vi "Lixiang's SRAM SEU mapping.vi"() -> ()   [LabVIEW 2015]
panel:
  out "subarray":i32[][](array[numeric])
  out "Array 2":i32[][](array[numeric])
  out "Intensity Graph 3":i32[][](graph)
  out "Intensity Graph 2":i32[][](graph)
  out "Intensity Graph":i32[][](graph)
  out "output array 3":bool[][](array[boolean])
  out "output array 2":bool[][](array[boolean])
  out "output array":bool[][](array[boolean])
  out "Array":u32[](array[numeric])
  out "number of replacements":i32
  out "SEU Information":string
  out "1->0":dbl
  out "0->1":dbl
  out "SEU":dbl
  in  "Data Pattern":i32=2
  out "result string":string
  out "text":string
  # "SRAM SEU Data Processing Program"
  # "Regular Model"
  # "0: 00  \n1: 10\n2: 11"
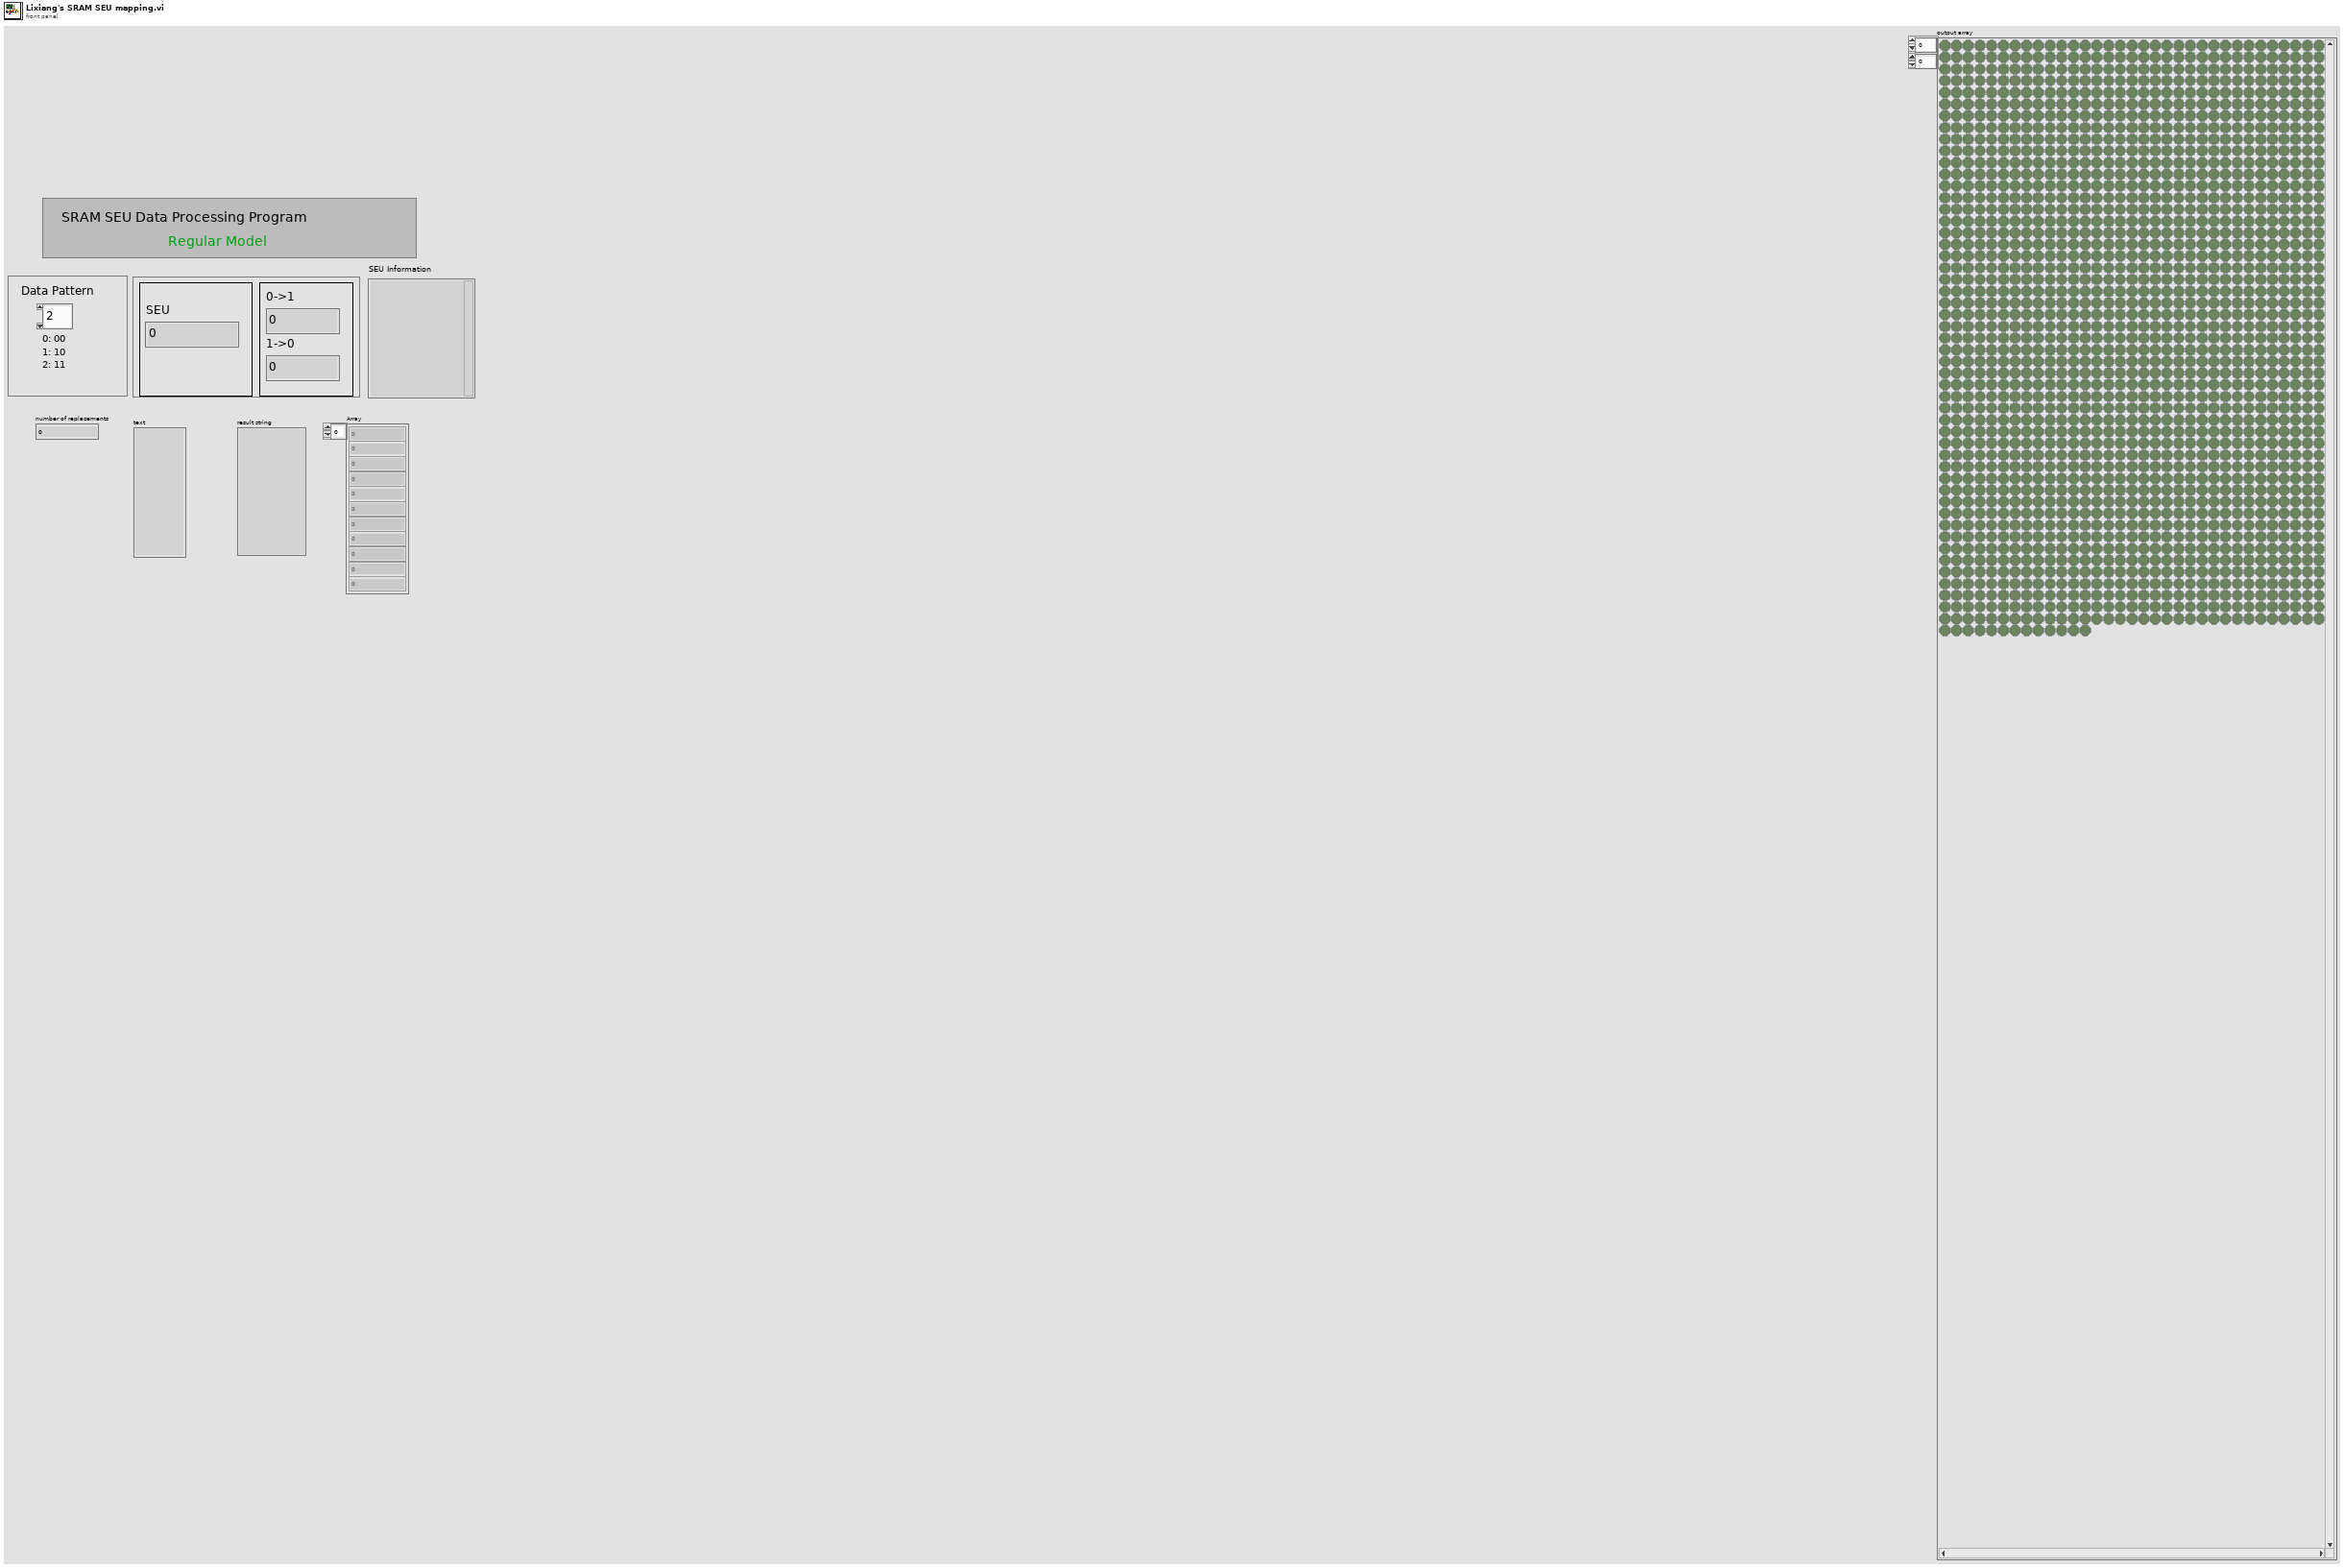
[diagram p1: front panel]
types:
  T1 = typedef "imagedata.ctl" = cluster{"image type":i32, "image depth":i32, "image":u8[], "mask":u8[], "colors":u32[], "Rectangle":cluster{"left":i16, "top":i16, "right":i16, "bottom":i16}}
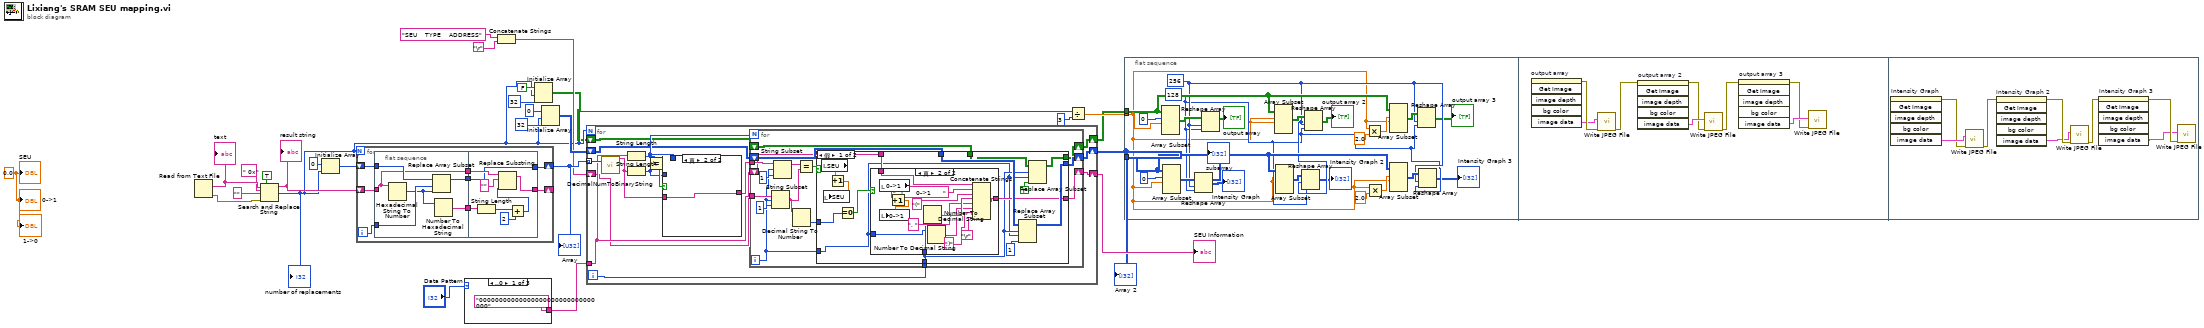
[diagram p0: block diagram]
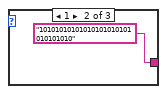
[diagram p2: hidden frame]
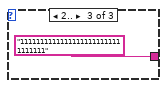
[diagram p3: hidden frame]
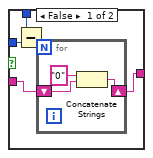
[diagram p4: hidden frame]
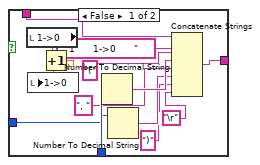
[diagram p5: hidden frame]
diagram:
  w16 = 0.0 ("Numeric 2")
  n1 = Read from Text File() -> (text=w27:string, error out=w24:errorcluster)  [unwired: 4 in, 2 out]
  "text" <- w27
  n2 = Search and Replace String(replace all?=TRUE ("replace all? (F)"), input string=w27, search string=" 0x", replace string="" ("replace string (\"\")"), error in=w24) -> (result string=w21:string, number of replacements=w4:i32)  [unwired: 3 in, 2 out]
  "result string" <- w21
  "number of replacements" <- w4
  n3 = Initialize Array(u32 0 ("element"), w4) -> (w20:u32[])
  n4 = for {
    N: w4 -> [_]
    shift-right: [w28] -> _
    shift-left: w21 -> [w35]
    shift-right: [w29] -> w19
    shift-left: w20 -> [w34]
    i -> [w33]
    n5 = flat-sequence {
      tunnel: w35 -> [w39]
      tunnel: w34 -> [w41]
      tunnel: w33 -> [w40]
      tunnel: [w39] -> w32
      tunnel: [w37] -> w31
      tunnel: [w36] -> w30
      tunnel: w32 -> [w49]
      tunnel: w31 -> [w47]
      tunnel: [w48] -> w29
      tunnel: w30 -> [w48]
      tunnel: [w45] -> w28
      frame #0 {
        n6 = Hexadecimal String To Number(string=w39) -> (number=w38:u32)  [unwired: 2 in, 1 out]
        n7 = Replace Array Subset(array=w41, new element=w38, index=w40) -> (w36:u32[])
        n8 = Number To Hexadecimal String(2:w38) -> (0:w37:string)  [unwired: 1 in]
      }
      frame #1 {
        n9 = String Length(string=w47) -> (length=w44:i32)
        n10 = Add(x=w44, y=u32 2) -> (x+y=w42:u32)
        n11 = Replace Substring(2:w42, 4:"" ("substring (\"\")"), 5:w49) -> (1:w45:string)  [unwired: 1 in, 1 out]
      }
    }
  }
  "Array" <- w19
  n12 = case shown="..0" "Data Pattern" {
    tunnel: ["00000000000000000000000000000000" "10101010101010101010101010101010" "11111111111111111111111111111111"] -> w17
    frame ..0 {
    }
    frame 1 {
    }
    frame 2.. {
    }
  }
  n13 = Concatenate Strings("SEU    TYPE    ADDRESS" ("string"), "\r") -> (w11:string)
  n14 = Initialize Array(FALSE, w4, 32 ("dimension size")) -> (w3:bool[][])
  n15 = Initialize Array(0, w4, 32 ("dimension size")) -> (w14:i32[][])
  n16 = for {
    N: w4 -> [_]
    tunnel: w19 -> [w66] mode=indexing
    tunnel: w17 -> [w65]
    shift-right: [w57] -> w7
    shift-left: w14 -> [w59]
    shift-right: [w55] -> w10
    shift-left: w11 -> [w56]
    shift-right: [w53] -> w1
    shift-left: w3 -> [w54]
    i -> [w58]
    n17 = call "DecimalNumToBinaryString.vi"("十进制 整形"=w66) -> ("二进制字符串"=w63:string)  [unwired: 10 in]
    n18 = String Length(string=w65) -> (length=w61:i32)
    n19 = String Length(string=w63) -> (length=w60:i32)
    n20 = Equal?(x=w61, y=w60) -> (x = y?=w64:bool)
    n21 = case shown="真" w64 {
      tunnel: w63 -> [w68 w75]
      tunnel: [w67 w75] -> w62
      tunnel: w61 -> [w71 _]
      tunnel: w60 -> [w70 _]
      frame False {
        n22 = Subtract(x=w71, y=w70) -> (x-y=w69:i32)
        n23 = for {
          N: w69 -> [_]
          shift-right: [w72] -> w67
          shift-left: w68 -> [w73]
          n24 = Concatenate Strings("0" ("string"), w73) -> (w72:string)
        }
      }
      frame True {
      }
    }
    n25 = for {
      N: w61 -> [_]
      tunnel: w62 -> [w91]
      tunnel: w65 -> [w87]
      tunnel: w58 -> [w83]
      shift-right: [w80] -> w57
      shift-left: w59 -> [w82]
      shift-right: [w78] -> w55
      shift-left: w56 -> [w79]
      shift-right: [w76] -> w53
      shift-left: w54 -> [w77]
      i -> [w81]
      n26 = String Subset(string=w87, offset (0)=w81, length (rest)=1 ("length (rest)")) -> (substring=w85:string)
      n27 = String Subset(string=w91, offset (0)=w81, length (rest)=1 ("length (rest)")) -> (substring=w90:string)
      n28 = Decimal String To Number(string=w85) -> (number=w84:i32)  [unwired: 2 in, 1 out]
      n29 = Equal?(x=w90, y=w85) -> (x = y?=w86:bool)
      n30 = case shown="假" w86 {
        tunnel: w84 -> [w103 _]
        tunnel: w83 -> [w93 _]
        tunnel: w82 -> [w101 w134]
        tunnel: w81 -> [w92 _]
        tunnel: [w100 w134] -> w80
        tunnel: w79 -> [w99 w133]
        tunnel: [w98 w133] -> w78
        tunnel: w77 -> [w95 w132]
        tunnel: [w94 w132] -> w76
        frame False {
          n31 = local read "SEU"() -> (w104:dbl)
          n32 = Increment(x=w104) -> (x+1=w105:dbl)
          n33 = local write "SEU"(w105) -> ()
          n34 = Equal To 0?(x=w103) -> (x = 0?=w102:bool)
          n35 = case shown="真" w102 {
            tunnel: w99 -> [w116 w124]
            tunnel: w93 -> [w113 w123]
            tunnel: w92 -> [w110 w122]
            tunnel: [w107 w121] -> w98
            frame False {
              n36 = local read "1->0"() -> (w117:dbl)
              n37 = Increment(x=w117) -> (x+1=w118:dbl)
              n38 = local write "1->0"(w118) -> ()
              n39 = Number To Decimal String(number=w113) -> (decimal integer string=w112:string)  [unwired: 1 in]
              n40 = Number To Decimal String(number=w110) -> (decimal integer string=w109:string)  [unwired: 1 in]
              n41 = Concatenate Strings(w116, "  1      1->0      " ("string"), "(" ("string"), w112, ", " ("string"), w109, ")" ("string"), "\r") -> (w107:string)
            }
            frame True {
              n42 = local read "0->1"() -> (w131:dbl)
              n43 = Increment(x=w131) -> (x+1=w130:dbl)
              n44 = local write "0->1"(w130) -> ()
              n45 = Number To Decimal String(number=w123) -> (decimal integer string=w128:string)  [unwired: 1 in]
              n46 = Number To Decimal String(number=w122) -> (decimal integer string=w126:string)  [unwired: 1 in]
              n47 = Concatenate Strings(w124, "  1      0->1      " ("string"), "(" ("string"), w128, ", " ("string"), w126, ")" ("string"), "\r") -> (w121:string)
            }
          }
          n48 = Replace Array Subset(array=w101, new element=1, index (row)=w93, index (col)=w92) -> (w100:i32[][])
          n49 = Replace Array Subset(array=w95, new element=TRUE, index (row)=w93, index (col)=w92) -> (w94:bool[][])
        }
        frame True {
        }
      }
    }
  }
  "SEU Information" <- w10
  "Array 2" <- w7
  n50 = Divide(x=w4, y=u32 3 ("dimension size")) -> (x/y=w2:dbl)
  n51 = flat-sequence {
    tunnel: w7 -> [w151]
    tunnel: w2 -> [w138]
    tunnel: w1 -> [w155]
    frame #0 {
      w139 = 128 ("dimension size")
      w140 = 256 ("dimension size")
      n52 = Array Subset(array=w155, index (row)=0 ("index"), length (row)=w138) -> (w149:bool[][])  [unwired: 2 in]
      n53 = Array Subset(array=w151, index (row)=0 ("index"), length (row)=w138) -> (w147:i32[][])  [unwired: 2 in]
      "subarray" <- w147
      n54 = Reshape Array(w147, w140, w139) -> (→"Intensity Graph":i32[][])
      n55 = Reshape Array(w149, w140, w139) -> (→"output array":bool[][])
      n56 = Array Subset(array=w155, index (row)=w138, length (row)=w138) -> (w145:bool[][])  [unwired: 2 in]
      n57 = Array Subset(array=w151, index (row)=w138, length (row)=w138) -> (w143:i32[][])  [unwired: 2 in]
      n58 = Reshape Array(w143, w140, w139) -> (→"Intensity Graph 2":i32[][])
      n59 = Reshape Array(w145, w140, w139) -> (→"output array 2":bool[][])
      n60 = Multiply(x=w138, y=2.0) -> (x*y=w150:dbl)
      n61 = Multiply(x=w138, y=2.0) -> (x*y=w154:dbl)
      n62 = Array Subset(array=w155, index (row)=w150, length (row)=w138) -> (w142:bool[][])  [unwired: 2 in]
      n63 = Array Subset(array=w151, index (row)=w154, length (row)=w138) -> (w141:i32[][])  [unwired: 2 in]
      n64 = Reshape Array(w142, w140, w139) -> (→"output array 3":bool[][])
      n65 = Reshape Array(w141, w140, w139) -> (→"Intensity Graph 3":i32[][])
    }
    frame #1 {
      n66 = invoke on="output array" class="Arr (strict)" method="Get Image"() -> (error out=w165:errorcluster, "image data"=w164:T1)  [unwired: 6 in, 4 out]
      n67 = call <vilib>:"Write JPEG File.vi"("error in (no error)"=w165, "image data"=w164) -> ("error out"=w162:errorcluster)  [unwired: 8 in, 1 out]
      n68 = invoke on="output array 2" class="Arr (strict)" method="Get Image"(error in=w162) -> (error out=w161:errorcluster, "image data"=w163:T1)  [unwired: 5 in, 4 out]
      n69 = call <vilib>:"Write JPEG File.vi"("error in (no error)"=w161, "image data"=w163) -> ("error out"=w160:errorcluster)  [unwired: 8 in, 1 out]
      n70 = invoke on="output array 3" class="Arr (strict)" method="Get Image"(error in=w160) -> (error out=w158:errorcluster, "image data"=w159:T1)  [unwired: 5 in, 4 out]
      n71 = call <vilib>:"Write JPEG File.vi"("error in (no error)"=w158, "image data"=w159) -> ()  [unwired: 8 in, 2 out]
    }
    frame #2 {
      n72 = invoke on="Intensity Graph" class="IntGraph (strict)" method="Get Image"() -> (error out=w166:errorcluster, "image data"=w167:T1)  [unwired: 6 in, 4 out]
      n73 = call <vilib>:"Write JPEG File.vi"("error in (no error)"=w166, "image data"=w167) -> ("error out"=w172:errorcluster)  [unwired: 8 in, 1 out]
      n74 = invoke on="Intensity Graph 2" class="IntGraph (strict)" method="Get Image"(error in=w172) -> (error out=w169:errorcluster, "image data"=w168:T1)  [unwired: 5 in, 4 out]
      n75 = call <vilib>:"Write JPEG File.vi"("error in (no error)"=w169, "image data"=w168) -> ("error out"=w173:errorcluster)  [unwired: 8 in, 1 out]
      n76 = invoke on="Intensity Graph 3" class="IntGraph (strict)" method="Get Image"(error in=w173) -> (error out=w171:errorcluster, "image data"=w170:T1)  [unwired: 5 in, 4 out]
      n77 = call <vilib>:"Write JPEG File.vi"("error in (no error)"=w171, "image data"=w170) -> ()  [unwired: 8 in, 2 out]
    }
  }
  "SEU" <- w16
  "0->1" <- w16
  "1->0" <- w16
